vi "Read.vi"(8 "error in (no error)":errorcluster, 9 "byte count":u32, 10 "Address":u8 format="%.0x", 11 "I2C Bus in":refnum<class "I2C Bus.lvclass">) -> (0 "error out":errorcluster, 2 "Data Out":u8[](array[numeric]) format="%.0x", 3 "I2C Bus out":refnum<class "I2C Bus.lvclass">)   [LabVIEW 2020, in "I2C Bus.lvclass"]
uses:
  I2C Bus.lvclass
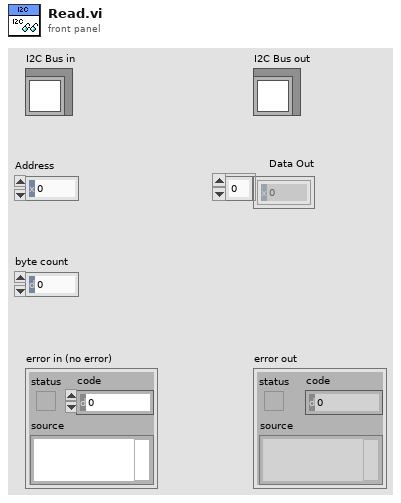
[diagram p1: front panel]
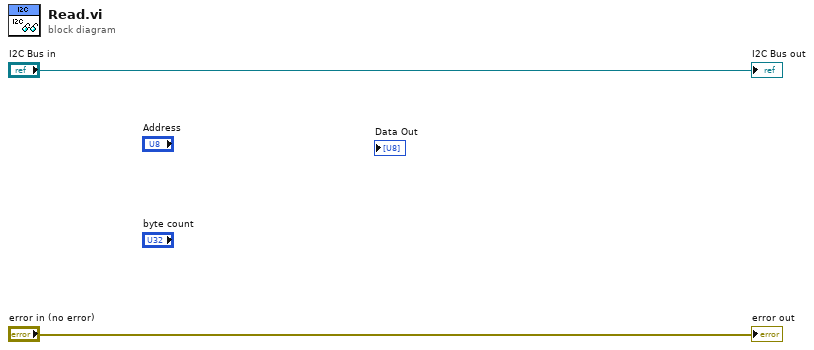
[diagram p0: block diagram]
diagram:
  "error out" <- "error in (no error)"
  "I2C Bus out" <- "I2C Bus in"
